vi "转换需保存的状态.vi"(2 "Container State":T1 caption="容器状态", 3 "Display State":T2={"完成"=FALSE, "功能选择"=enum."扫描", "数据"=[], "历史数据"=[], "曲线设置"={"X"=enum."设置电压", "Y1"=enum."读取电流", "Y2"=enum."无", "Y3"=enum."无"}, "突变电压"=refnum, "保留数量"=0} caption="显示状态") -> (1 "Display State To Save":variant caption="待保存显示状态")   [LabVIEW 2020, in "数据显示.xctl"]
uses:
  <vilib>/_xctls/Container State.ctl
  <vilib>/_xctls/XControlSupport.lvlib
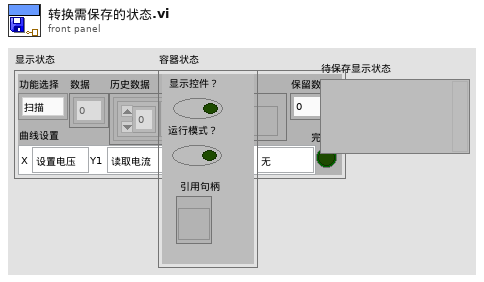
[diagram p1: front panel]
types:
  T1 = typedef "XControlSupport.lvlib/Container State.ctl" = cluster{"Indicator?":bool, "Run Mode?":bool, " Refnum":refnum<vi>}
  T2 = typedef "数据显示.xctl/状态.ctl" = cluster{"完成":bool, "功能选择":enum16{"扫描", "循环扫描", "保持时间", "脉冲", "高速脉冲", "任意波形"}, "数据":dbl[][], "历史数据":T3[], "曲线设置":T4, "突变电压":refnum<user-event>, "保留数量":i32}
  T3 = typedef "数据显示.xctl/波形数据定义.ctl" = cluster{"波形":dbl[][], "属性":variant}
  T4 = typedef "数据显示.xctl/曲线设置.ctl" = cluster{"X":enum16{"时间", "设置电压", "读取电流", "读取电压"}, "Y1":enum16{"时间", "设置电压", "读取电流", "读取电压"}, "Y2":enum16{"时间", "设置电压", "读取电流", "读取电压", "无"}, "Y3":enum16{"时间", "设置电压", "读取电流", "读取电压", "无"}}
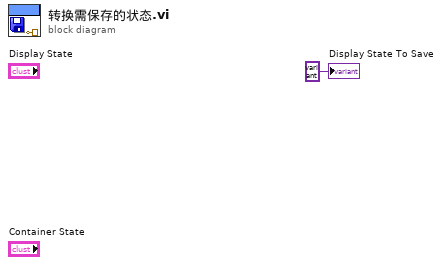
[diagram p0: block diagram]
diagram:
  "Display State To Save" <- variant ("Display State To Save")
